vi "publisehr tests 2.vi"() -> ()   [LabVIEW 2018]
uses:
  publisher action.ctl
  <vilib>/ActorFramework/Reply Msg/Reply Msg.lvclass
panel:
  out "Numeric":i32
  out "number":dbl
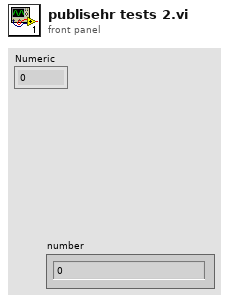
[diagram p1: front panel]
types:
  T1 = typedef "publisher action.ctl" = enum16{"set", "get", "init", "--send request", "--wait", "--respond", "init writer", "init reader"}
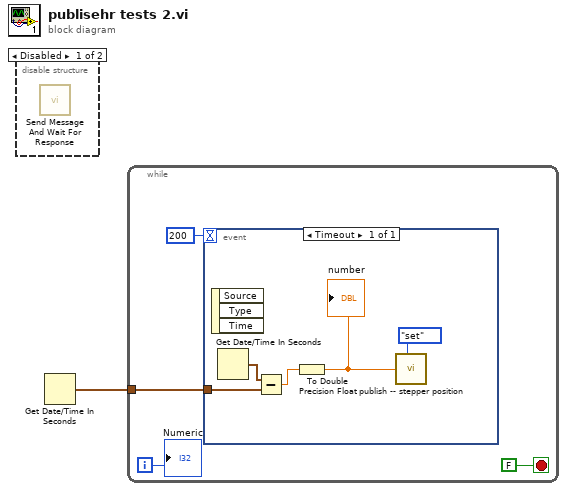
[diagram p0: block diagram]
diagram:
  n1 = disable-structure shown="Disabled" {
    frame Disabled {
      n2 = call <vilib>:"Send Message And Wait For Response.vi"() -> ()  [unwired: 8 in, 4 out]
    }
    frame Enabled {
    }
  }
  n3 = Get Date/Time In Seconds() -> (seconds since 1Jan1904=w1:timestamp)
  n4 = while {
    tunnel: w1 -> [w2]
    i -> [w3]
    stop <- FALSE stop-if-true
    n5 = event shown="[0] Timeout" {
      selector: _ -> [_]
      dyn-events: _ -> [_]
      timeout: 200 -> [_]
      tunnel: w2 -> [w6]
      event Timeout {
        n6 = event-data() -> ()  [unwired: 1 in, 3 out]
        n7 = Get Date/Time In Seconds() -> (seconds since 1Jan1904=w8:timestamp)
        n8 = Subtract(x=w8, y=w6) -> (x-y=w7:dbl)
        n9 = To Double Precision Float(number=w7) -> (double precision float=w9:dbl)
        "number" <- w9
        n10 = call "publish -- stepper position.vi"("publisher action"=publisher_action."set", "stepper pos IN"=w9) -> ()  [unwired: 9 in, 1 out]
      }
    }
    "Numeric" <- w3
  }
